vi "Read Header Content.vi"(8 "error in (no error)":errorcluster, 11 "Simulated_Header in":refnum<class "Simulated_Header.lvclass">) -> (0 "error out":errorcluster, 2 "Header Content":string[][](array[string]), 3 "Simulated_Header out":refnum<class "Simulated_Header.lvclass">)   [LabVIEW 2018, in "Simulated_Header.lvclass"]
uses:
  Simulated_Header.lvclass
  Simulated_Header.lvclass/Simulated_Header.ctl
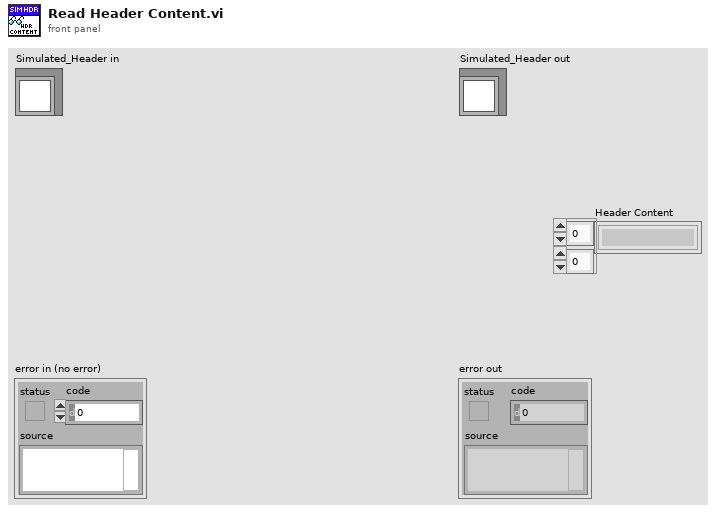
[diagram p1: front panel]
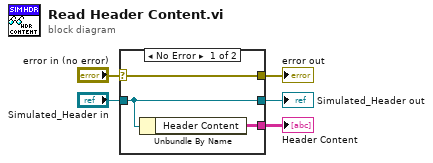
[diagram p0: block diagram]
diagram:
  n1 = case shown="No Error" "error in (no error)" {
    selector: "error in (no error)" -> [w8 w9]
    tunnel: [w8 w9] -> w4
    tunnel: [w7 w10] -> w2
    tunnel: "Simulated_Header in" -> [w7 w10]
    tunnel: [w6 _] -> w1
    frame No Error {
      n2 = Unbundle By Name(w7) -> ("Header Content"=w6:string[][])
    }
    frame Error {
    }
  }
  "error out" <- w4
  "Simulated_Header out" <- w2
  "Header Content" <- w1
